vi "Call EDS Read.vi"(11 "SDO Parameters":T1 {"Block Data" format="%.0x"}) -> (3 "SDO Parameters out":T1 {"Block Data" format="%.0x"})   [LabVIEW 2021, in "CANOpen Addon System Explorer.lvlib"]
uses:
  CANOpen Addon System Explorer.lvlib
  Shared/SDO Parameters Array.ctl
  Shared/CANOpen_SDO Settings.ctl
  Shared/CANOpen Addon Shared.lvlib
panel:
  # "LSB"
  # "MSB"
  # "LSB"
  # "MSB"
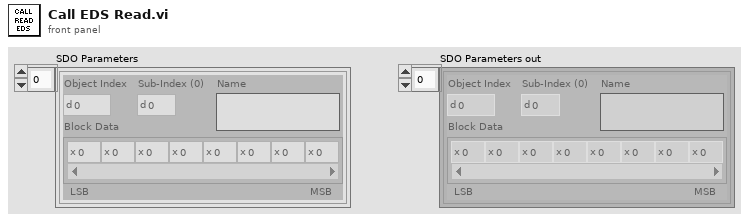
[diagram p1: front panel]
types:
  T1 = typedef "CANOpen Addon Shared.lvlib/SDO Parameters Array.ctl" = T2[]
  T2 = typedef "CANOpen Addon Shared.lvlib/CANOpen_SDO Settings.ctl" = cluster{"Object Index":u16, "Sub-Index (0)":u8, "Block Data":u8[], "Name":string}
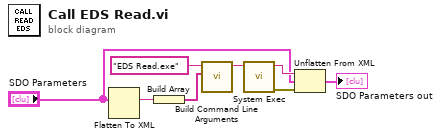
[diagram p0: block diagram]
diagram:
  n1 = Flatten To XML(6:"SDO Parameters") -> (2:w4:string)
  n2 = Build Array(w4) -> (w6:string[])
  n3 = call "Build Command Line Arguments.vi"("Arguments"=w6, "Executable File Name"="EDS Read.exe") -> ("Command Line"=w5:string)  [unwired: 9 in]
  n4 = call <vilib>:"System Exec.vi"("command line"=w5) -> ("error out"=w7:errorcluster, "standard output"=w3:string)  [unwired: 7 in, 2 out]
  n5 = Unflatten From XML(xml string=w3, type="SDO Parameters", error in (no error)=w7) -> (value=→"SDO Parameters out":T1)  [unwired: 1 out]
